vi "FB Switch Input Term No Var.vi"(8 "error in":errorcluster, 11 "data in":variant) -> (0 "error out":errorcluster, 3 "data out":variant)   [LabVIEW 2017]
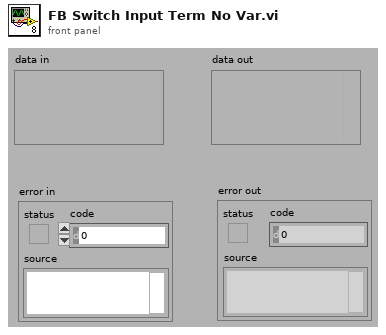
[diagram p1: front panel]
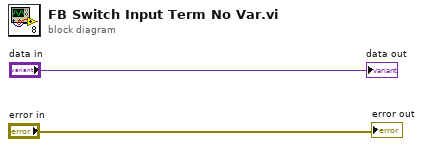
[diagram p0: block diagram]
diagram:
  "data out" <- "data in"
  "error out" <- "error in"
